vi "multiplier.vi"() -> ()   [LabVIEW 2014]
panel:
  out "XY^2-1":dbl
  in  "Y":dbl
  in  "X":dbl
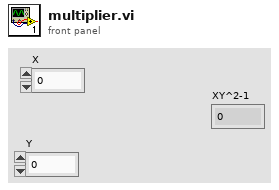
[diagram p1: front panel]
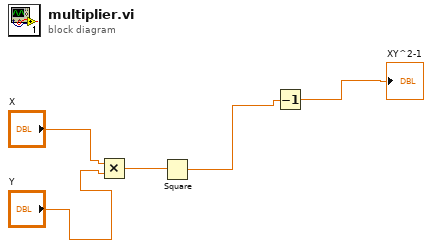
[diagram p0: block diagram]
diagram:
  n1 = Multiply(x="X", y="Y") -> (x*y=w3:dbl)
  n2 = Square(x=w3) -> (x^2=w2:dbl)
  n3 = Decrement(x=w2) -> (x-1=→"XY^2-1":dbl)
